vi "op_num_v7.vi"() -> ()   [LabVIEW 2009]
panel:
  out "Gr":dbl
  out "A":dbl
  out "V":dbl
  out "Cos fi":dbl
  out "Sin fi":dbl
  in  "Unghiul de dafazaj gr":dbl(knob) scale=0.0..90.0
  out "Paparenta - W":dbl
  out "P reactiva - W":dbl
  out "Pa -Kw":dbl(knob) scale=0.0..15.0
  out "Pr-Kw":dbl(knob) scale=0.0..15.0
  out "P activa - W":dbl
  out "P -Kw":dbl(knob) scale=0.0..15.0
  in  "Curent -A":dbl(knob) scale=0.0..50.0
  in  "Tensiune - V":dbl(knob) scale=0.0..250.0
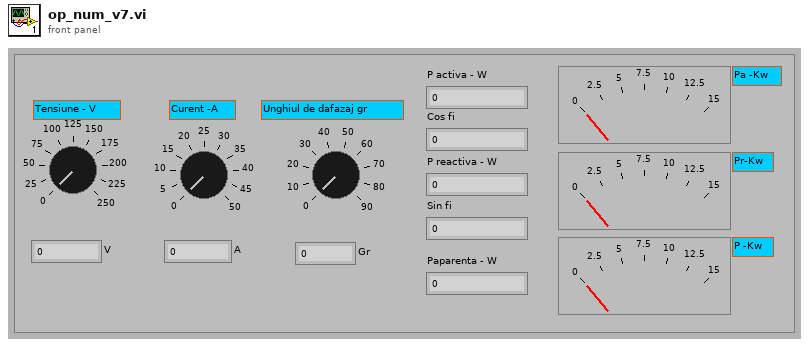
[diagram p1: front panel]
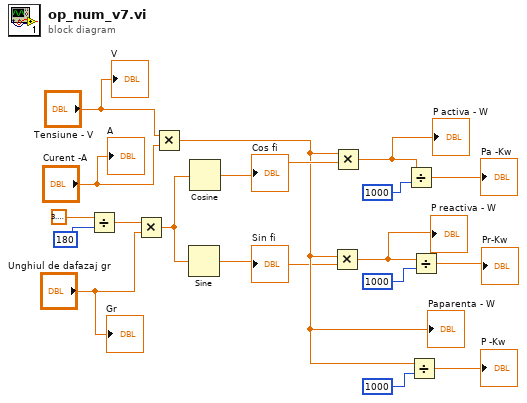
[diagram p0: block diagram]
diagram:
  n1 = Divide(x=3.141592653589793, y=180) -> (x/y=w15:dbl)
  n2 = Multiply(x=w15, y="Unghiul de dafazaj gr") -> (x*y=w14:dbl)
  n3 = Multiply(x="Tensiune - V", y="Curent -A") -> (x*y=w9:dbl)
  "Paparenta - W" <- w9
  n4 = Sine(x=w14) -> (sin(x)=w8:dbl)
  "Sin fi" <- w8
  n5 = Cosine(x=w14) -> (cos(x)=w13:dbl)
  "Cos fi" <- w13
  n6 = Multiply(x=w9, y=w8) -> (x*y=w4:dbl)
  "P reactiva - W" <- w4
  n7 = Multiply(x=w9, y=w13) -> (x*y=w10:dbl)
  "P activa - W" <- w10
  n8 = Divide(x=w10, y=1000) -> (x/y=→"Pa -Kw":dbl)
  n9 = Divide(x=w9, y=1000) -> (x/y=→"P -Kw":dbl)
  n10 = Divide(x=w4, y=1000) -> (x/y=→"Pr-Kw":dbl)
  "V" <- "Tensiune - V"
  "A" <- "Curent -A"
  "Gr" <- "Unghiul de dafazaj gr"
